vi "grSim Packet Command UDP.vi"(5 "grSim Port":u16=20011, 7 "grSim IP Address":string="127.0.0.1", 8 "error in":errorcluster, 10 "Blue Robots":T1[](array[typedef]), 11 "Yellow Robots":T1[](array[typedef])) -> (0 "error out":errorcluster)   [LabVIEW 2016]
uses:
  grSim Robot Command.ctl
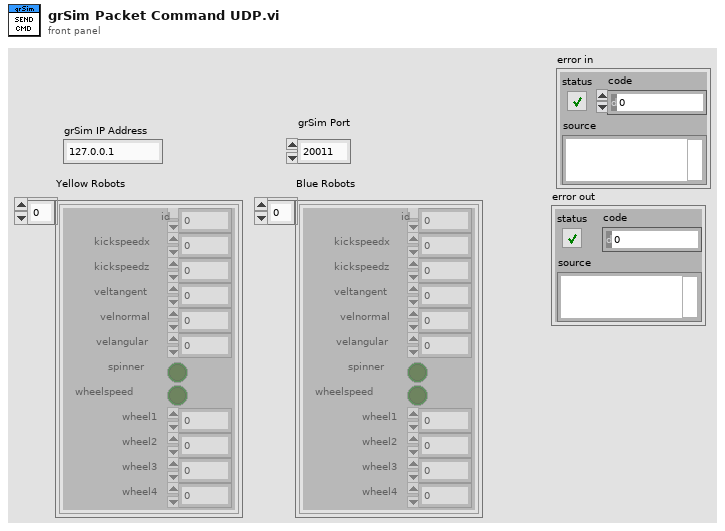
[diagram p1: front panel]
types:
  T1 = typedef "grSim Robot Command.ctl" = cluster{"id":u32, "kickspeedx":sgl, "kickspeedz":sgl, "veltangent":sgl, "velnormal":sgl, "velangular":sgl, "spinner":bool, "wheelspeed":bool, "wheel1":sgl, "wheel2":sgl, "wheel3":sgl, "wheel4":sgl}
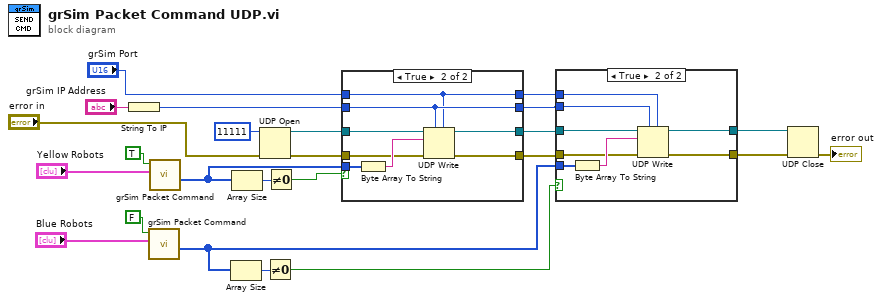
[diagram p0: block diagram]
diagram:
  n1 = String To IP(1:"grSim IP Address") -> (0:w15:u32)
  n2 = call "grSim Packet Command.vi"("Robots"="Blue Robots", "isteamyellow"=FALSE) -> ("Array"=w4:u8[])  [unwired: 9 in]
  n3 = call "grSim Packet Command.vi"("Robots"="Yellow Robots", "isteamyellow"=TRUE) -> ("Array"=w16:u8[])  [unwired: 9 in]
  n4 = Array Size(array=w4) -> (size(s)=w5:i32)
  n5 = Array Size(array=w16) -> (size(s)=w18:i32)
  n6 = UDP Open(8:"error in", 11:u16 11111 ("port")) -> (port=w13:refnum<k16>, 0:w14:errorcluster)  [unwired: 3 in, 1 out]
  n7 = Not Equal To 0?(x=w5) -> (x != 0?=w3:bool)
  n8 = Not Equal To 0?(x=w18) -> (x != 0?=w17:bool)
  n9 = case shown="True" w17 {
    tunnel: w16 -> [_ w36]
    tunnel: w15 -> [w26 w30]
    tunnel: w14 -> [w27 w34]
    tunnel: w13 -> [w28 w33]
    tunnel: [w28 w32] -> w12
    tunnel: [w27 w31] -> w11
    tunnel: [w26 w30] -> w8
    tunnel: "grSim Port" -> [w25 w29]
    tunnel: [w25 w29] -> w6
    frame False {
    }
    frame True {
      n10 = Byte Array To String(unsigned byte array=w36) -> (string=w35:string)
      n11 = UDP Write(address=w30, port or service name=w29, connection ID=w33, data in=w35, 8:w34) -> (error out=w31:errorcluster, 3:w32:refnum<k16>)  [unwired: 1 in]
    }
  }
  n12 = case shown="True" w3 {
    tunnel: w4 -> [_ w46]
    tunnel: w8 -> [_ w44]
    tunnel: w11 -> [w37 w43]
    tunnel: w12 -> [w38 w42]
    tunnel: [w38 w41] -> w10
    tunnel: [w37 w40] -> w9
    tunnel: w6 -> [_ w39]
    frame False {
    }
    frame True {
      n13 = Byte Array To String(unsigned byte array=w46) -> (string=w45:string)
      n14 = UDP Write(address=w44, port or service name=w39, connection ID=w42, data in=w45, 8:w43) -> (error out=w40:errorcluster, 3:w41:refnum<k16>)  [unwired: 1 in]
    }
  }
  n15 = UDP Close(connection ID=w10, 8:w9) -> (error out=→"error out":errorcluster)  [unwired: 1 out]
